vi "DMM Read Temperature.vi"() -> ()   [LabVIEW 2011]
uses:
  <instrlib>/DMM4/DMM4.lvlib
panel:
  in  "Simulation Value":dbl=23.0 min=0.0 max=50.0 step=0.01 format="%#.2f"
  in  "Temperature Unit":u16(ring) items=["C", "F"]
  in  "Type for Temperature":u16(ring) items=["J Type", "K Type", "T Type"]
  out "error out":errorcluster
  out "Measure Value":string
  in  "Stop":bool
  out "Boolean":bool
  in  "Detector Rate":u16(ring) items=["SLOW", "MID", "FAST"]
  out "ID Return String":string
  in  "Configure RS232 Baud Rate":u32(ring)=115200 items=["9600"=9600, "19200"=19200, "38400"=38400, "57600"=57600, "115200"=115200]
  in  "VISA resource name":refnum<visa-resource-name>
  # "DMM Read Temperature"
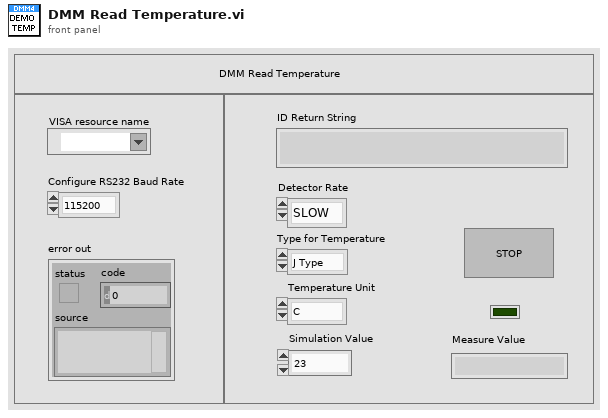
[diagram p1: front panel]
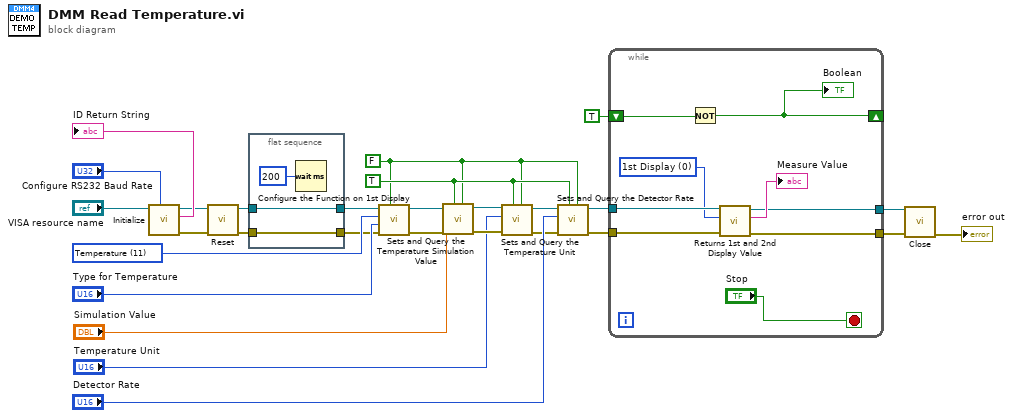
[diagram p0: block diagram]
diagram:
  w7 = FALSE ("Enable to Query")
  w8 = TRUE ("Enable to Sets")
  w25 = u8 11 items=["DC Voltage", "AC Voltage", "DC+AC Voltage", "DC Current", "AC Current", "DC+AC Current", "2-Wire Resistance", "Frequency", "Period", "Continuity", "Diode", "Temperature", "Capacitance"] ("Function")
  n1 = call <instrlib>:"Initialize.vi"("Configure RS232 Baud Rate"="Configure RS232 Baud Rate", "VISA resource name"="VISA resource name") -> ("error out"=w17:errorcluster, "ID Return String"=→"ID Return String":string, "VISA resource name out"=w18:refnum<visa-resource-name>)  [unwired: 6 in, 1 out]
  n2 = call <instrlib>:"Reset.vi"("error in (no error)"=w17, "VISA resource name"=w18) -> ("error out"=w2:errorcluster, "VISA resource name out"=w4:refnum<visa-resource-name>)  [unwired: 8 in]
  n3 = flat-sequence {
    tunnel: w4 -> [w31]
    tunnel: [w31] -> w3
    tunnel: w2 -> [w30]
    tunnel: [w30] -> w1
    frame #0 {
      n4 = Wait (ms)(milliseconds to wait=u32 200) -> ()  [unwired: 1 out]
    }
  }
  n5 = call <instrlib>:"Configure the Function on 1st Display .vi"("Enable Auto Range"=w7, "error in"=w1, "Type for Temperature"="Type for Temperature", "Function"=w25, "VISA resource name"=w3) -> ("error out"=w10:errorcluster, "VISA resource name out"=w12:refnum<visa-resource-name>)  [unwired: 5 in]
  n6 = call <instrlib>:"Sets and Query the Temperature Simulation Value.vi"("Enable to Query"=w7, "Enable to Sets"=w8, "error in"=w10, "Simulation Value"="Simulation Value", "VISA resource name"=w12) -> ("error out"=w9:errorcluster, "VISA resource name out"=w11:refnum<visa-resource-name>)  [unwired: 4 in, 1 out]
  n7 = call <instrlib>:"Sets and Query the Temperature Unit.vi"("Enable to Query"=w7, "Enable to Sets"=w8, "error in"=w9, "Temperature Unit"="Temperature Unit", "VISA resource name"=w11) -> ("error out"=w14:errorcluster, "VISA resource name out"=w13:refnum<visa-resource-name>)  [unwired: 4 in, 1 out]
  n8 = call <instrlib>:"Sets and Query the Detector Rate.vi"("Enable to Query"=w7, "Enable to Sets"=w8, "error in"=w14, "Detector Rate"="Detector Rate", "VISA resource name"=w13) -> ("error out"=w22:errorcluster, "VISA resource name out"=w23:refnum<visa-resource-name>)  [unwired: 4 in, 1 out]
  n9 = while {
    tunnel: w23 -> [w40]
    tunnel: w22 -> [w39]
    tunnel: [w35] -> w21
    tunnel: [w34] -> w20
    shift-right: [w32] -> _
    shift-left: TRUE -> [w33]
    stop <- "Stop" stop-if-true
    w38 = u16 0 items=["1st Display", "2nd Display", "1st & 2nd Display"] ("Sets to Display")
    n10 = Not(x=w33) -> (.not. x?=w32:bool)
    "Boolean" <- w32
    n11 = call <instrlib>:"Returns 1st and 2nd Display Value.vi"("error in"=w39, "Sets to Display"=w38, "VISA resource name"=w40) -> ("error out"=w34:errorcluster, "Return the Value"=→"Measure Value":string, "VISA resource name out"=w35:refnum<visa-resource-name>)  [unwired: 6 in]
  }
  n12 = call <instrlib>:"Close.vi"("error in (no error)"=w20, "VISA resource name"=w21) -> ("error out"=→"error out":errorcluster)  [unwired: 9 in]
